vi "SNTP Light RT Driver VI_SNTP Part_Moving Averaging.vi"(8 "error in (no error)":errorcluster, 11 "Last Offset Value":dbl) -> (0 "error in (no error) 2":errorcluster, 3 "Averaged Value":dbl)   [LabVIEW 2013]
uses:
  <vilib>/ptbypt/NI_PtbyPt.lvlib
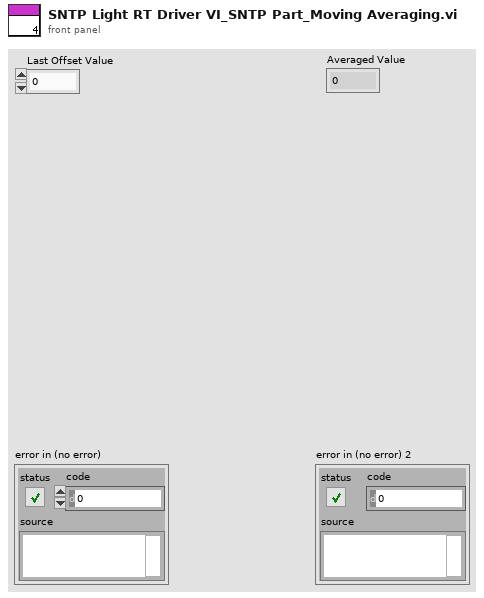
[diagram p1: front panel]
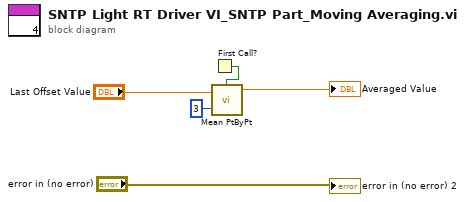
[diagram p0: block diagram]
diagram:
  n1 = First Call?() -> (First Call?: T/F=w1:bool)
  n2 = call <vilib>:"Mean PtByPt.vi"("x"="Last Offset Value", "sample length"=3, "initialize"=w1) -> ("mean"=→"Averaged Value":dbl)  [unwired: 1 in, 1 out]
  "error in (no error) 2" <- "error in (no error)"
